vi "SCLN_ExampleOneServerWithParser.vi"() -> ()   [LabVIEW 2015]
uses:
  SCLN_RW_Select.ctl
panel:
  in  "Power Switch":bool
  in  "Temperature":dbl(slide) scale=0.0..100.0
  out "Conn1":bool
  out "Loop1":i32=1
  out "error out":errorcluster
  in  "Config filename":path=path "C:/soar/comm/SCLN/config/soar_comms.cfg"
  in  "stop":bool
  out "Message Out":string
  out "Message In":string="ERROR SERVER SHUTDOWN"
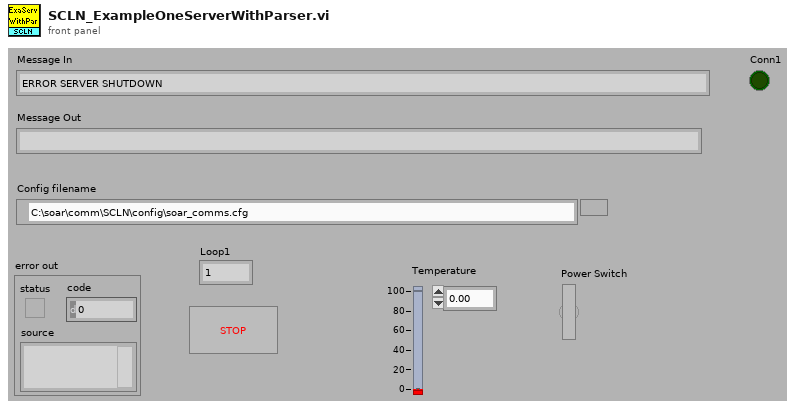
[diagram p1: front panel]
types:
  T1 = typedef "SCLN_RW_Select.ctl" = enum16{"Read", "Write"}
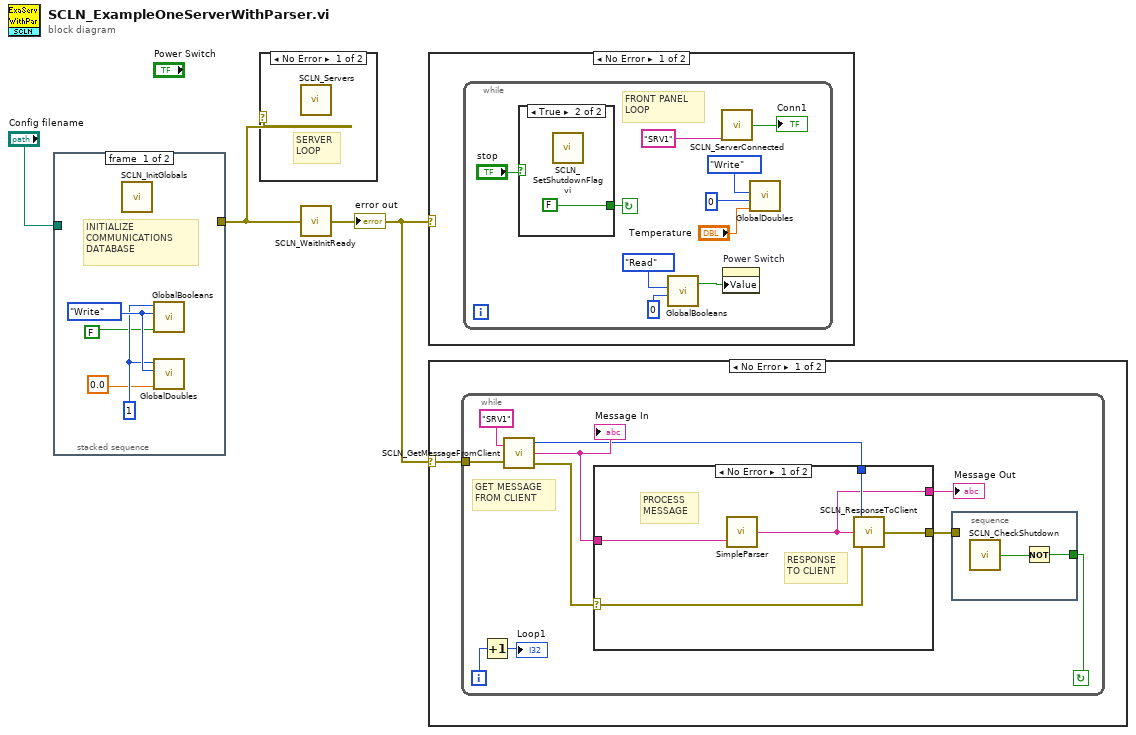
[diagram p0: block diagram]
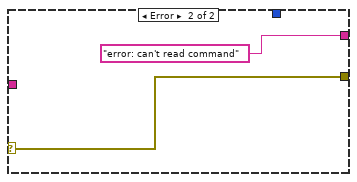
[diagram p2: hidden frame]
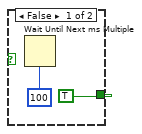
[diagram p4: hidden frame]
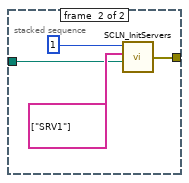
[diagram p7: hidden frame]
diagram:
  n1 = stacked-sequence {
    tunnel: "Config filename" -> [_ w9]
    tunnel: [_ w8] -> w2
    frame #0 {
      w6 = 1
      w7 = SCLN_RW_Select."Write" ("GBL_RW")
      # "INITIALIZE\nCOMMUNICATIONS\nDATABASE"
      n2 = call "SCLN_InitGlobals.vi"() -> ()  [unwired: 1 in]
      n3 = call "GlobalBooleans.vi"("Write Value"=FALSE, "Operation"=w7, "Number of Elements"=w6) -> ()  [unwired: 1 in, 2 out]
      n4 = call "GlobalDoubles.vi"("Write Value"=0.0, "Operation"=w7, "Number of elements"=w6) -> ()  [unwired: 1 in, 2 out]
    }
    frame #1 {
      n5 = call "SCLN_InitServers.vi"("Config File Name"=w9, "Server Names"=string[] ["SRV1"], "Num of Servers"=1) -> ("error out"=w8:errorcluster)  [unwired: 1 in]
    }
  }
  n6 = case shown="No Error" w2 {
    frame No Error {
      # "SERVER\nLOOP"
      n7 = call "SCLN_Servers.vi"() -> ()  [unwired: 1 out]
    }
    frame Error {
    }
  }
  n8 = call "SCLN_WaitInitReady.vi"("error in (no error)"=w2) -> ("error out"=w1:errorcluster)
  "error out" <- w1
  n9 = case shown="No Error" w1 {
    frame No Error {
      n10 = while {
        stop <- w20 continue-if-true
        # "FRONT PANEL\nLOOP"
        n11 = case shown="True" "stop" {
          tunnel: [TRUE FALSE] -> w20
          frame False {
            n12 = Wait Until Next ms Multiple(millisecond multiple=100) -> ()  [unwired: 1 out]
          }
          frame True {
            n13 = call "SCLN_SetShutdownFlagvi.vi"() -> ()  [unwired: 1 in]
          }
        }
        n14 = call "GlobalBooleans.vi"("Element"=0, "Operation"=SCLN_RW_Select."Read" ("GBL_RW")) -> ("Read Value"=w12:bool)  [unwired: 2 in, 1 out]
        n15 = call "SCLN_ServerConnected.vi"("Server Name"="SRV1") -> ("Connected"=→"Conn1":bool)
        n16 = property on="Power Switch" class="Bool (strict)"("Value"=w12) -> ()  [unwired: 2 in, 2 out]
        n17 = call "GlobalDoubles.vi"("Write Value"="Temperature", "Element"=0, "Operation"=SCLN_RW_Select."Write" ("GBL_RW")) -> ()  [unwired: 1 in, 2 out]
      }
    }
    frame Error {
    }
  }
  n18 = case shown="No Error" w1 {
    selector: w1 -> [w25 _]
    frame No Error {
      n19 = while {
        tunnel: w25 -> [w34]
        i -> [w28]
        stop <- w30 continue-if-true
        # "GET MESSAGE\nFROM CLIENT"
        n20 = Increment(x=w28) -> (x+1=→"Loop1":i32)
        n21 = call "SCLN_GetMessageFromClient.vi"("Server Name"="SRV1", "error in (no error)"=w34) -> ("Index for Response"=w32:i32, "Message"=w33:string, "error out"=w27:errorcluster)
        "Message In" <- w33
        n22 = case shown="No Error" w27 {
          selector: w27 -> [w40 w44]
          tunnel: w33 -> [w39 _]
          tunnel: w32 -> [w42 _]
          tunnel: [w41 w44] -> w31
          tunnel: [w38 "error: can't read command" ("time string")] -> w26
          frame No Error {
            # "PROCESS\nMESSAGE"
            # "RESPONSE\nTO CLIENT"
            n23 = call "SimpleParser.vi"("Command"=w39) -> ("Response"=w38:string)
            n24 = call "SCLN_ResponseToClient.vi"("error in (no error)"=w40, "Message"=w38, "Index for Response"=w42) -> ("error out"=w41:errorcluster)
          }
          frame Error {
          }
        }
        "Message Out" <- w26
        n25 = stacked-sequence {
          tunnel: [w36] -> w30
          tunnel: w31 -> [_]
          frame #0 {
            n26 = call "SCLN_CheckShutdown.vi"() -> ("Shutdown"=w37:bool)
            n27 = Not(x=w37) -> (.not. x?=w36:bool)
          }
        }
      }
    }
    frame Error {
    }
  }
